vi "parte_2.vi"(11 "info":i32) -> (2 "pin_int":i32, 3 "pin_string":string)   [LabVIEW 2021]
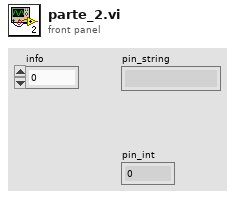
[diagram p1: front panel]
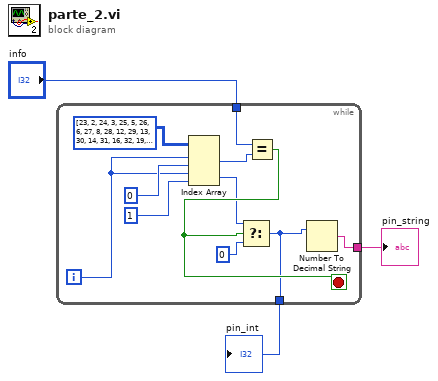
[diagram p0: block diagram]
diagram:
  n1 = while {
    tunnel: "info" -> [w13]
    tunnel: [w6] -> w3
    tunnel: [w5] -> w2
    i -> [w10]
    stop <- w9 stop-if-true
    n2 = Index Array(array=i32[][] [[23, 2], [24, 3], [25, 5], [26, 6], [27, 8], [28, 12], [29, 13], [30, 14], [31, 16], [32, 19], [33, 20], [34, 21], [35, 22], [36, 23], [37, 27], [38, 28], [39, 29], [40, 30], [41, 31], [42, 32], [43, 33], [44, 34], [45, 36], [46, 37], [47, 38], [48, 39], [49, 40], [50, 41], [51, 42], [52, 43], [53, 44]], index (row) #1=w10, index (col) #1=0 ("index (row)"), index (row) #2=w10, index (col) #2=1 ("index (row)")) -> (element #1=w14:i32, element #2=w8:i32)
    n3 = Equal?(x=w13, y=w14) -> (x = y?=w9:bool)
    n4 = Select(t=w8, s=w9, f=0) -> (s? t:f=w6:i32)
    n5 = Number To Decimal String(number=w6) -> (decimal integer string=w5:string)  [unwired: 1 in]
  }
  "pin_int" <- w3
  "pin_string" <- w2
